vi "Guitar Subvi2.vi"(0 "error out":errorcluster, 1 "Image Dst Out":T1, 2 "Blue Guitar 2":T2={"Global Rectangle"=[569, 290, 594, 372], "Contours"=[{"ID"=enum."External", "Type"=2, "Coordinates"=[593, 371, 569, 290]}]} {"Contours"."Type" items=["No Selection", "Point", "Line", "Rectangle", "Oval", "Polygon", "Freehand Region", "Annulus", "Unused2", "Unused3", "Broken Line", "Freehand Line", "Rotated Rectangle"]}, 3 "Yellow Guitar 2":T2={"Global Rectangle"=[546, 282, 563, 376], "Contours"=[{"ID"=enum."External", "Type"=2, "Coordinates"=[562, 375, 546, 282]}]} {"Contours"."Type" items=["No Selection", "Point", "Line", "Rectangle", "Oval", "Polygon", "Freehand Region", "Annulus", "Unused2", "Unused3", "Broken Line", "Freehand Line", "Rotated Rectangle"]}, 4 "Green Guitar 2":T2={"Global Rectangle"=[498, 284, 505, 376], "Contours"=[{"ID"=enum."External", "Type"=2, "Coordinates"=[498, 375, 504, 284]}]} {"Contours"."Type" items=["No Selection", "Point", "Line", "Rectangle", "Oval", "Polygon", "Freehand Region", "Annulus", "Unused2", "Unused3", "Broken Line", "Freehand Line", "Rotated Rectangle"]}, 5 "Red Guitar 2":T2={"Global Rectangle"=[526, 284, 530, 370], "Contours"=[{"ID"=enum."External", "Type"=2, "Coordinates"=[529, 369, 526, 284]}]} {"Contours"."Type" items=["No Selection", "Point", "Line", "Rectangle", "Oval", "Polygon", "Freehand Region", "Annulus", "Unused2", "Unused3", "Broken Line", "Freehand Line", "Rotated Rectangle"]}, 6 "Orange Guitar 2":T2={"Global Rectangle"=[587, 282, 628, 378], "Contours"=[{"ID"=enum."External", "Type"=2, "Coordinates"=[627, 377, 587, 282]}]} {"Contours"."Type" items=["No Selection", "Point", "Line", "Rectangle", "Oval", "Polygon", "Freehand Region", "Annulus", "Unused2", "Unused3", "Broken Line", "Freehand Line", "Rotated Rectangle"]}) -> (11 "Orange Guitar LED":bool, 13 "Red Guitar LED":bool, 15 "Green Guitar LED":bool, 23 "Blue Guitar LED":bool, 24 "Yellow Guitar LED":bool, 27 "error out 2":errorcluster)   [LabVIEW 2009]
uses:
  <vilib>/vision/Image Controls.llb/IMAQ Image.ctl
  <vilib>/Analysis/3filter.llb/Filter Passband Type.ctl
  <vilib>/Analysis/3filter.llb/Butterworth Filter (DBL).vi
  <vilib>/Analysis/NI_AALBase.lvlib
  <vilib>/vision/NI_Vision_Development_Module.lvlib
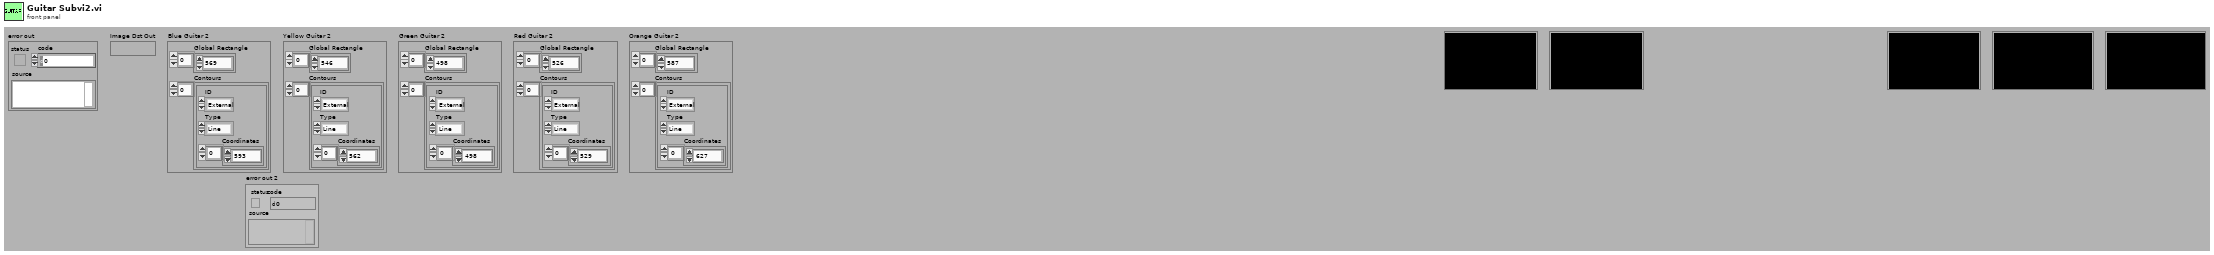
[diagram p1: front panel]
types:
  T1 = typedef "IMAQ Image.ctl" = refnum<image>
  T2 = cluster{"Global Rectangle":i32[], "Contours":cluster{"ID":enum32{"External", "Internal"}, "Type":u32, "Coordinates":i32[]}[]}
  T3 = typedef "NI_AALBase.lvlib/Filter Passband Type.ctl" = enum32{"Lowpass", "Highpass", "Bandpass", "Bandstop"}
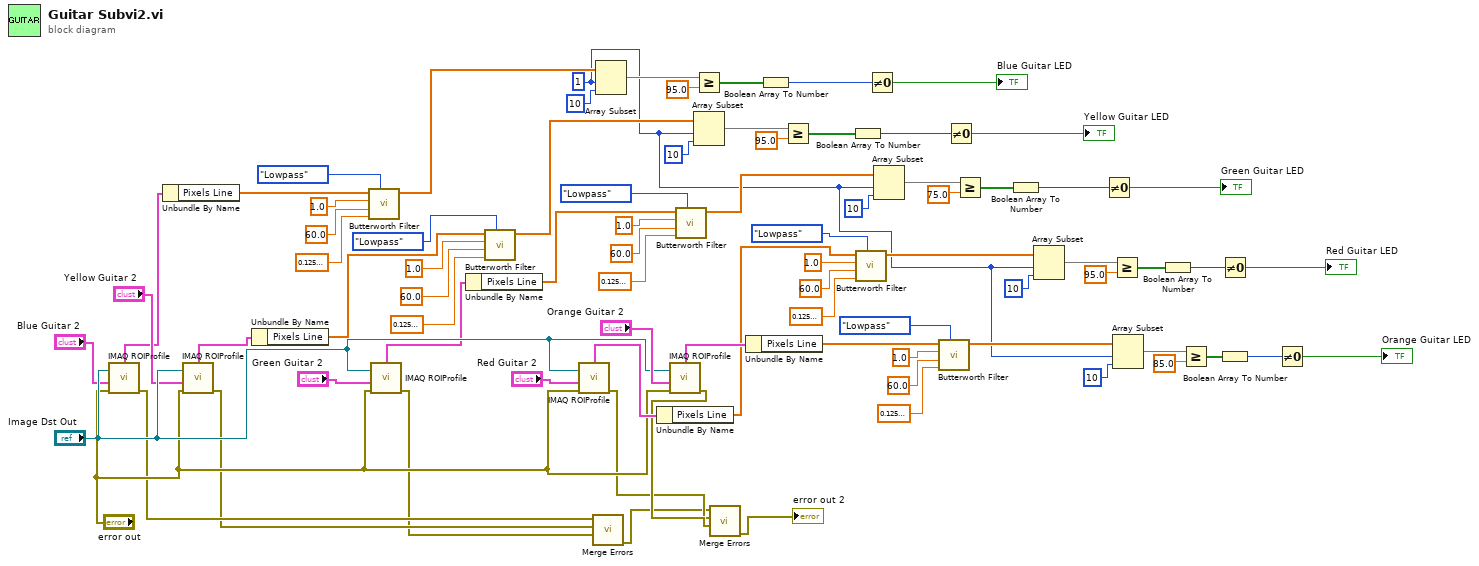
[diagram p0: block diagram]
diagram:
  w9 = 1 ("index")
  n1 = call "IMAQ ROIProfile"("error in (no error)"="error out", "ROI Descriptor"="Blue Guitar 2", "Image"="Image Dst Out") -> ("error out"=w6:errorcluster, "ROI Graph"=w47:cluster{"x0":sgl, "dx":sgl, "Pixels Line":sgl[]})  [unwired: 4 out]
  n2 = Unbundle By Name(w47) -> ("Pixels Line"=w67:sgl[])
  n3 = call "IMAQ ROIProfile"("error in (no error)"="error out", "ROI Descriptor"="Yellow Guitar 2", "Image"="Image Dst Out") -> ("error out"=w5:errorcluster, "ROI Graph"=w50:cluster{"x0":sgl, "dx":sgl, "Pixels Line":sgl[]})  [unwired: 4 out]
  n4 = Unbundle By Name(w50) -> ("Pixels Line"=w53:sgl[])
  n5 = call-poly <vilib>:"Butterworth Filter.vi"("filter type"=Filter_Passband_Type."Lowpass", "low cutoff freq: fl"=0.12500000000000006 ("low 3"), "high cutoff freq: fh"=60.0 ("high 14"), "sampling freq: fs"=1.0 ("sampling  9"), "X"=w67) -> ("Filtered X"=w34:dbl[])  [unwired: 3 in, 1 out]
  n6 = call "IMAQ ROIProfile"("error in (no error)"="error out", "ROI Descriptor"="Green Guitar 2", "Image"="Image Dst Out") -> ("error out"=w4:errorcluster, "ROI Graph"=w45:cluster{"x0":sgl, "dx":sgl, "Pixels Line":sgl[]})  [unwired: 4 out]
  n7 = Unbundle By Name(w45) -> ("Pixels Line"=w42:sgl[])
  n8 = call-poly <vilib>:"Butterworth Filter.vi"("filter type"=Filter_Passband_Type."Lowpass", "low cutoff freq: fl"=0.12500000000000006 ("low  12"), "high cutoff freq: fh"=60.0 ("high 13"), "sampling freq: fs"=1.0 ("sampling 12"), "X"=w53) -> ("Filtered X"=w49:dbl[])  [unwired: 3 in, 1 out]
  n9 = call "IMAQ ROIProfile"("error in (no error)"="error out", "ROI Descriptor"="Red Guitar 2", "Image"="Image Dst Out") -> ("error out"=w2:errorcluster, "ROI Graph"=w23:cluster{"x0":sgl, "dx":sgl, "Pixels Line":sgl[]})  [unwired: 4 out]
  n10 = call <vilib>:"Merge Errors.vi"("error in 3 (no error)"=w4, "error in 2 (no error)"=w5, "error in 1 (no error)"=w6) -> ("error out"=w1:errorcluster)  [unwired: 4 in]
  n11 = Array Subset(array=w34, index=w9, length=10) -> (w62:dbl[])
  n12 = Unbundle By Name(w23) -> ("Pixels Line"=w26:sgl[])
  n13 = call "IMAQ ROIProfile"("error in (no error)"="error out", "ROI Descriptor"="Orange Guitar 2", "Image"="Image Dst Out") -> ("error out"=w3:errorcluster, "ROI Graph"=w74:cluster{"x0":sgl, "dx":sgl, "Pixels Line":sgl[]})  [unwired: 4 out]
  n14 = call-poly <vilib>:"Butterworth Filter.vi"("filter type"=Filter_Passband_Type."Lowpass", "low cutoff freq: fl"=0.12500000000000006 ("low  11"), "high cutoff freq: fh"=60.0 ("high 12"), "sampling freq: fs"=1.0 ("sampling 11"), "X"=w42) -> ("Filtered X"=w46:dbl[])  [unwired: 3 in, 1 out]
  n15 = Greater Or Equal?(x=w62, y=95.0) -> (x >= y?=w10:bool[])
  n16 = Array Subset(array=w49, index=w9, length=10) -> (w58:dbl[])
  n17 = call <vilib>:"Merge Errors.vi"("error in 3 (no error)"=w3, "error in 2 (no error)"=w2, "error in 1 (no error)"=w1) -> ("error out"=→"error out 2":errorcluster)  [unwired: 4 in]
  n18 = Unbundle By Name(w74) -> ("Pixels Line"=w18:sgl[])
  n19 = Boolean Array To Number(Boolean array=w10) -> (number=w60:u32)
  n20 = Greater Or Equal?(x=w58, y=95.0) -> (x >= y?=w56:bool[])
  n21 = Boolean Array To Number(Boolean array=w56) -> (number=w55:u32)
  n22 = call-poly <vilib>:"Butterworth Filter.vi"("filter type"=Filter_Passband_Type."Lowpass", "low cutoff freq: fl"=0.12500000000000006 ("low  10"), "high cutoff freq: fh"=60.0 ("high 11"), "sampling freq: fs"=1.0 ("sampling 10"), "X"=w26) -> ("Filtered X"=w22:dbl[])  [unwired: 3 in, 1 out]
  n23 = Not Equal To 0?(x=w60) -> (x != 0?=→"Blue Guitar LED":bool)
  n24 = Array Subset(array=w46, index=w9, length=10) -> (w37:dbl[])
  n25 = call-poly <vilib>:"Butterworth Filter.vi"("filter type"=Filter_Passband_Type."Lowpass", "low cutoff freq: fl"=0.12500000000000006 ("low  9"), "high cutoff freq: fh"=60.0 ("high 10"), "sampling freq: fs"=1.0 ("sampling 9"), "X"=w18) -> ("Filtered X"=w21:dbl[])  [unwired: 3 in, 1 out]
  n26 = Not Equal To 0?(x=w55) -> (x != 0?=→"Yellow Guitar LED":bool)
  n27 = Greater Or Equal?(x=w37, y=75.0) -> (x >= y?=w39:bool[])
  n28 = Boolean Array To Number(Boolean array=w39) -> (number=w40:u32)
  n29 = Array Subset(array=w22, index=w9, length=10) -> (w31:dbl[])
  n30 = Not Equal To 0?(x=w40) -> (x != 0?=→"Green Guitar LED":bool)
  n31 = Greater Or Equal?(x=w31, y=95.0) -> (x >= y?=w29:bool[])
  n32 = Array Subset(array=w21, index=w9, length=10) -> (w13:dbl[])
  n33 = Boolean Array To Number(Boolean array=w29) -> (number=w28:u32)
  n34 = Greater Or Equal?(x=w13, y=85.0) -> (x >= y?=w15:bool[])
  n35 = Not Equal To 0?(x=w28) -> (x != 0?=→"Red Guitar LED":bool)
  n36 = Boolean Array To Number(Boolean array=w15) -> (number=w16:u32)
  n37 = Not Equal To 0?(x=w16) -> (x != 0?=→"Orange Guitar LED":bool)
